vi "Update Tree Item Icon.vi"(0 "TreeControl in":refnum<vi>, 5 "Measurement folder Tags":string[](array[string]), 7 "Measurement file Tags":string[](array[string]), 9 "Icon":i32, 11 "error in (no error)":errorcluster) -> (4 "TreeControl out":refnum<vi>, 15 "error out":errorcluster)   [LabVIEW 2021, in "Converter.lvlib"]
uses:
  Converter.lvlib
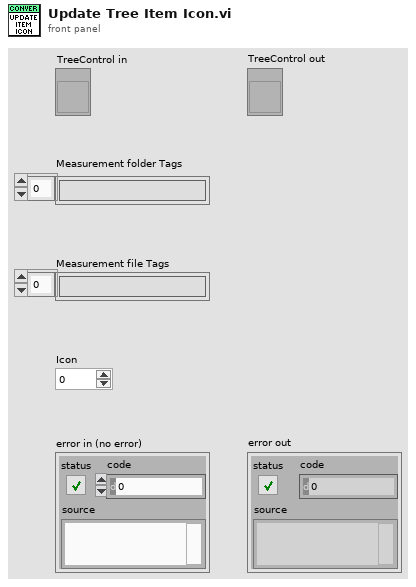
[diagram p1: front panel]
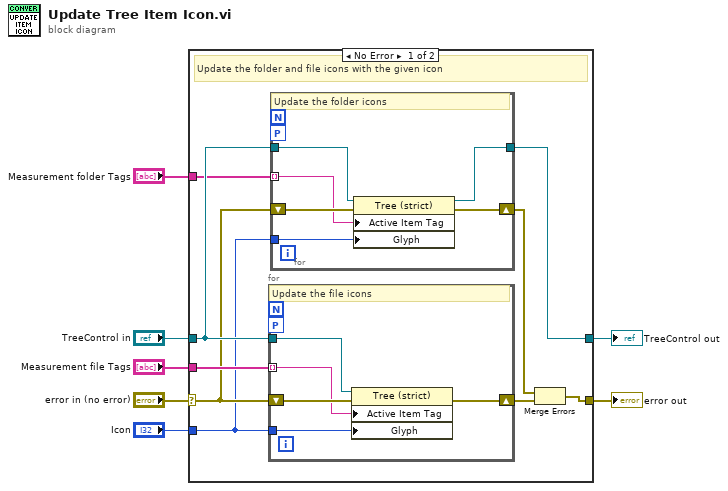
[diagram p0: block diagram]
diagram:
  n1 = case shown="No Error" "error in (no error)" {
    selector: "error in (no error)" -> [w13 w29]
    tunnel: "Measurement file Tags" -> [w16 _]
    tunnel: "TreeControl in" -> [w15 w28]
    tunnel: "Measurement folder Tags" -> [w14 _]
    tunnel: "Icon" -> [w12 _]
    tunnel: [w9 w29] -> w2
    tunnel: [w8 w28] -> w1
    frame No Error {
      # "Update the folder and file icons with the given icon"
      n2 = for {
        shift-right: [w26] -> w10
        shift-left: w13 -> [w27]
        workers-P: _ -> [_]
        tunnel: w16 -> [w25] mode=indexing
        tunnel: w12 -> [w24]
        tunnel: w15 -> [w23]
        # "Update the file icons"
        n3 = property on="Property Node" class="Tree (strict)"(reference=w23, error in=w27, "Active Item Tag"=w25, "Glyph"=w24) -> (error out=w26:errorcluster)  [unwired: 1 out]
      }
      n4 = for {
        shift-right: [w21] -> w11
        shift-left: w13 -> [w22]
        workers-P: _ -> [_]
        tunnel: w14 -> [w20] mode=indexing
        tunnel: w12 -> [w19]
        tunnel: w15 -> [w18]
        tunnel: [w17] -> w8
        # "Update the folder icons"
        n5 = property on="Property Node" class="Tree (strict)"(reference=w18, error in=w22, "Active Item Tag"=w20, "Glyph"=w19) -> (reference out=w17:refnum<vi>, error out=w21:errorcluster)
      }
      n6 = Merge Errors(w11, w10) -> (w9:errorcluster)
    }
    frame Error {
      # "Pass"
    }
  }
  "error out" <- w2
  "TreeControl out" <- w1
